vi "clLabview_BDPW_calcSalt.vi"(0 "vi_lib.lvlib:clLabview.lvclass":refnum<class "clLabview.lvclass">, 3 "MD5 password":string, 4 "Hash 1":string) -> (14 "Salt":string, 15 "Found Salt":bool)   [LabVIEW 2011, in "vi_lib.lvlib" / "clLabview.lvclass"]
uses:
  clLabview.lvclass
  vi_lib.lvlib
  clFileReader/clFileReader.lvclass
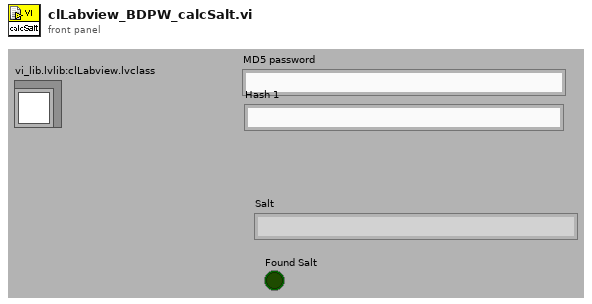
[diagram p1: front panel]
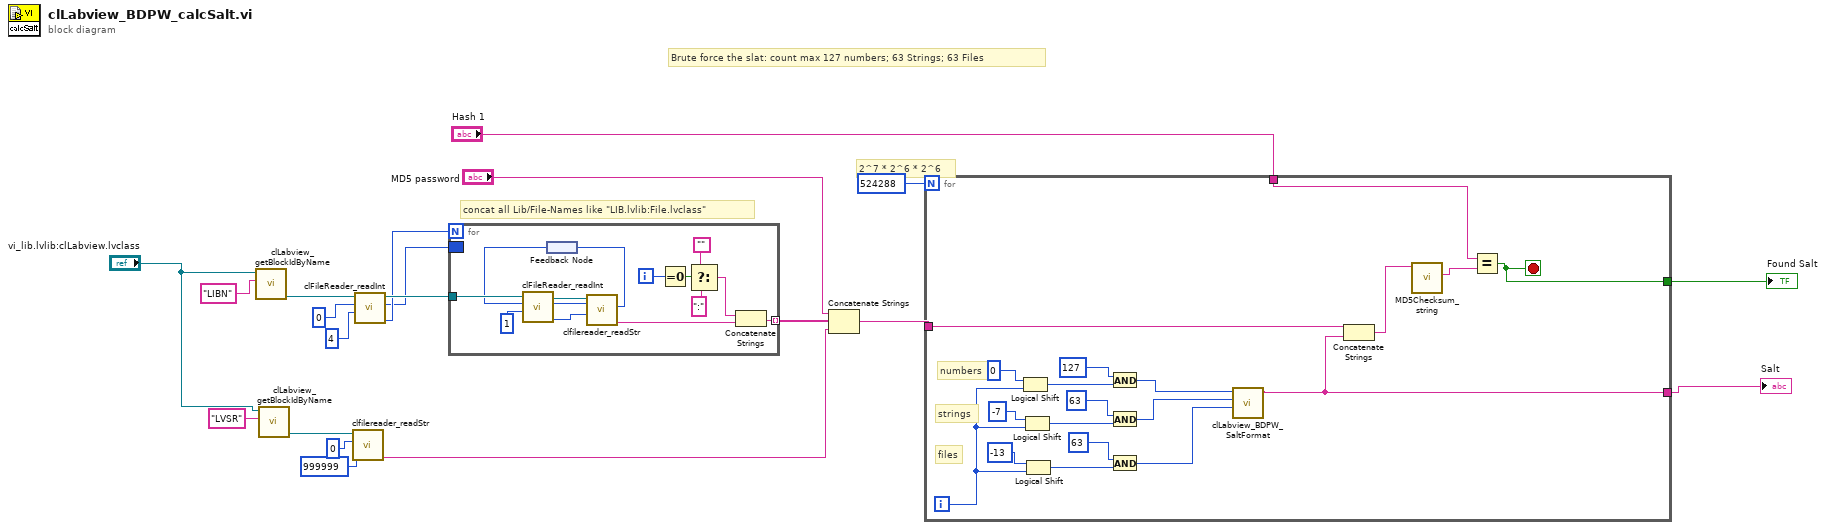
[diagram p0: block diagram]
diagram:
  # "concat all Lib/File-Names like \"LIB.lvlib:File.lvclass\""
  # "Brute force the slat: count max 127 numbers; 63 Strings; 63 Files"
  # "2^7 * 2^6 * 2^6"
  n1 = call "clLabview_getBlockIdByName.vi"("Block Name"="LIBN", "vi_lib.lvlib:clLabview.lvclass"="vi_lib.lvlib:clLabview.lvclass") -> ("Block Content"=w18:refnum<class "clFileReader.lvclass">)  [unwired: 2 in, 6 out]
  n2 = call "clLabview_getBlockIdByName.vi"("Block Name"="LVSR", "vi_lib.lvlib:clLabview.lvclass"="vi_lib.lvlib:clLabview.lvclass") -> ("Block Content"=w14:refnum<class "clFileReader.lvclass">)  [unwired: 2 in, 6 out]
  n3 = call "clfilereader_readStr.vi"("size"=u32 999999, "offset"=u32 0, "clFileReader.lvclass IN"=w14) -> ("ReadStr - OUT Value"=w11:string)  [unwired: 8 out]
  n4 = call "clFileReader_readInt.vi"("size"=u32 4, "offset"=u32 0, "clFileReader.lvclass IN"=w18) -> ("OUT Value"=w3:u32, "new offset"=w1:u32, "clFileReader.lvclass OUT"=w4:refnum<class "clFileReader.lvclass">)  [unwired: 6 out]
  n5 = for {
    N: w3 -> [_]
    tunnel: w4 -> [w34]
    tunnel: [w26] -> w15 mode=indexing
    border: w1 -> [_]
    i -> [w25]
    n6 = feedback #1() -> (w28:u32)
    n7 = call "clFileReader_readInt.vi"("size"=u32 1, "offset"=w28, "clFileReader.lvclass IN"=w34) -> ("OUT Value"=w30:u32, "new offset"=w31:u32, "clFileReader.lvclass OUT"=w32:refnum<class "clFileReader.lvclass">)  [unwired: 6 out]
    n8 = call "clfilereader_readStr.vi"("size"=w30, "offset"=w31, "clFileReader.lvclass IN"=w32) -> ("ReadStr - OUT Value"=w27:string, "new offset"=w29:u32)  [unwired: 7 out]
    n9 = feedback-in #1(w29) -> ()
    n10 = Equal To 0?(x=w25) -> (x = 0?=w24:bool)
    n11 = Select(t="", s=w24, f=":" ("ReadStr - OUT Value")) -> (s? t:f=w23:string)
    n12 = Concatenate Strings(w23, w27) -> (w26:string)
  }
  n13 = Concatenate Strings("MD5 password", w15, w11) -> (w8:string)
  n14 = for {
    N: u32 524288 ("size") -> [_]
    tunnel: w8 -> [w53]
    tunnel: "Hash 1" -> [w52]
    tunnel: [w42] -> w6
    tunnel: [w37] -> w5
    i -> [w48]
    stop <- w42 stop-if-true
    # "files"
    # "strings"
    # "numbers"
    n15 = Logical Shift(y=i8 0, x=w48) -> (x << y=w51:i32)
    n16 = Logical Shift(y=i8 -7, x=w48) -> (x << y=w49:i32)
    n17 = Logical Shift(y=i8 -13, x=w48) -> (x << y=w50:i32)
    n18 = And(x=127, y=w51) -> (x .and. y?=w40:i32)
    n19 = And(x=63, y=w49) -> (x .and. y?=w39:i32)
    n20 = And(x=63, y=w50) -> (x .and. y?=w38:i32)
    n21 = call "clLabview_BDPW_SaltFormat.vi"("count Path"=w38, "count String"=w39, "count Numeric"=w40) -> ("Salt"=w37:string)  [unwired: 8 out]
    n22 = Concatenate Strings(w53, w37) -> (w43:string)
    n23 = call "MD5Checksum_string.vi"("Message String"=w43) -> ("MD5 message-digest (Ascii)"=w41:string)  [unwired: 10 out]
    n24 = Equal?(x=w52, y=w41) -> (x = y?=w42:bool)
  }
  "Salt" <- w5
  "Found Salt" <- w6
